vi "Html Title Size.vi"(9 "字体大小":dbl) -> (1 "数值":dbl)   [LabVIEW 2014]
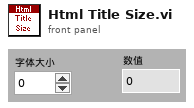
[diagram p1: front panel]
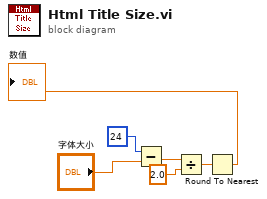
[diagram p0: block diagram]
diagram:
  n1 = Subtract(x=24, y="字体大小") -> (x-y=w2:dbl)
  n2 = Divide(x=w2, y=2.0) -> (x/y=w1:dbl)
  n3 = Round To Nearest(number=w1) -> (nearest integer value=→"数值":dbl)
